vi "DeActivate Panel Updates Poly.vi"   [LabVIEW 2023]
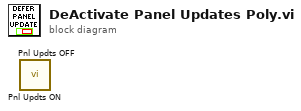
[diagram p0: block diagram]
diagram:
  n1 = call "Pnl Updts ON.vi"() -> ()  [unwired: 11 in, 1 out]
  n2 = call "Pnl Updts OFF.vi"() -> ()  [unwired: 11 in, 1 out]
